vi "MX100 Open Connection.vi"(8 "error in (no error)":errorcluster, 11 "Host Address (\"192.168.1.1\")":string="172.16.90.100") -> (0 "error out":errorcluster, 2 "MX100 Cluster":T1={"Base Time"=0, "Session Number"=0, "Last Data Number"={"High"=-1, "Low"=4294967295}, "Channel List"=[], "FIFO Number (0)"=0, "Channel Number (1)"=1, "Select FIFO or Channel (F:Channel)"=FALSE, "MX100 Data"={"Measurement Values out"=[], "Date/Time"=""}} {"Channel Number (1)" min=1 max=60 step=1; "FIFO Number (0)" min=-1 max=2 step=1}, 3 "VISA Refnum out":refnum<visa-resource-name>)   [LabVIEW 2016]
uses:
  Type Definitions/MX100 Initialization.ctl
  Type Definitions/MX100 Data.ctl
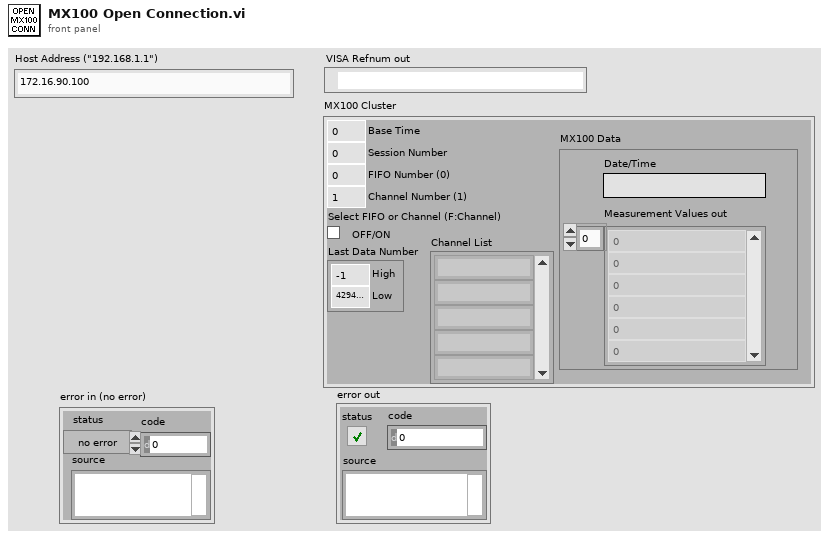
[diagram p1: front panel]
types:
  T1 = typedef "MX100 Initialization.ctl" = cluster{"Base Time":i32, "Session Number":i32, "Last Data Number":cluster{"High":i32, "Low":u32}, "Channel List":string[], "FIFO Number (0)":i32, "Channel Number (1)":i32, "Select FIFO or Channel (F:Channel)":bool, "MX100 Data":T2}
  T2 = typedef "MX100 Data.ctl" = cluster{"Measurement Values out":dbl[], "Date/Time":string}
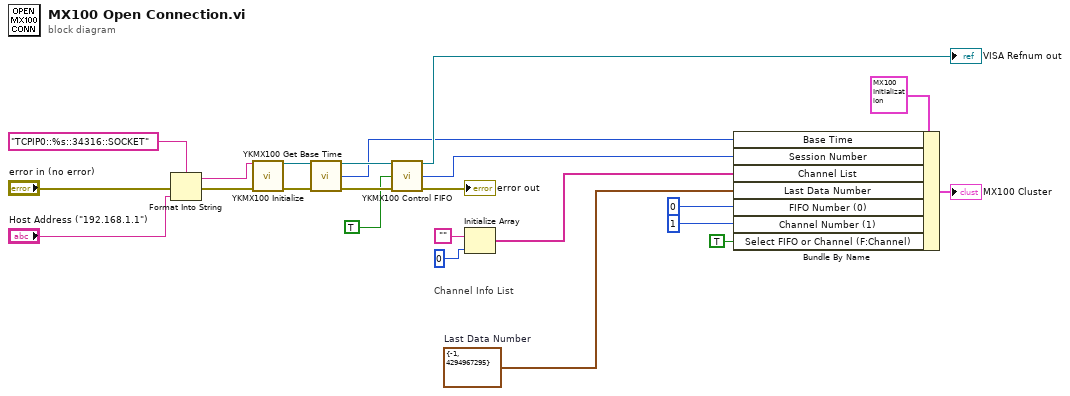
[diagram p0: block diagram]
diagram:
  w5 = cluster{"High":i32, "Low":u32} {"High"=-1, "Low"=4294967295}  # Last Data Number
  # "Channel Info List"
  n1 = Format Into String(format string="TCPIP0::%s::34316::SOCKET", error in="error in (no error)", "Host Address (\"192.168.1.1\")") -> (resulting string=w1:string, error out=w16:errorcluster)  [unwired: 1 in]
  n2 = call "YKMX100 Initialize.vi"("VISA session (TCPIP::)"=w1, "error in (no error)"=w16) -> ("dup VISA session"=w20:refnum<visa-resource-name>, "error out"=w22:errorcluster)  [unwired: 12 in]
  n3 = call "YKMX100 Get Base Time.vi"("VISA session"=w20, "error in (no error)"=w22) -> ("dup VISA session"=w21:refnum<visa-resource-name>, "Base Time"=w8:i32, "error out"=w23:errorcluster)  [unwired: 11 in]
  n4 = call "YKMX100 Control FIFO.vi"("VISA session"=w21, "FIFO (T:Start)"=TRUE, "error in (no error)"=w23) -> ("dup VISA session"=→"VISA Refnum out":refnum<visa-resource-name>, "Session Number"=w7:i32, "error out"=→"error out":errorcluster)  [unwired: 10 in]
  n5 = Initialize Array("", 0) -> (w6:string[])
  n6 = Bundle By Name(cluster=T1 {"Base Time"=0, "Session Number"=0, "Last Data Number"={"High"=-1, "Low"=4294967295}, "Channel List"=[], "FIFO Number (0)"=0, "Channel Number (1)"=1, "Select FIFO or Channel (F:Channel)"=FALSE, "MX100 Data"={"Measurement Values out"=[], "Date/Time"=""}} ("MX100 Cluster 2"), "Base Time"=w8, "Session Number"=w7, "Channel List"=w6, "Last Data Number"=w5, "FIFO Number (0)"=0, "Channel Number (1)"=1, "Select FIFO or Channel (F:Channel)"=TRUE) -> (→"MX100 Cluster":T1)
